vi "Untitled 1.vi"() -> ()   [LabVIEW 2015]
uses:
  <vilib>/Analysis/3filter.llb/Filter Passband Type.ctl
  <vilib>/Analysis/3filter.llb/Butterworth Filter (DBL).vi
  <vilib>/Analysis/NI_AALBase.lvlib
panel:
  in  "frequency":dbl=0.0078125 format="%0.4e"
  in  "amplitude 2":dbl=1.0 format="%0.2f"
  out "Waveform Graph":dbl[][](graph)
  out "Waveform Chart":dbl[](graph)
  in  "amplitude":dbl=1.0 format="%0.2f"
  in  "Cutoff 1":dbl=0.12500000000000006 format="%0.4f"
  in  "Cutoff 2":dbl=0.45000000000000007 format="%0.2f"
  in  "sampling freq: fs":dbl=1.0 format="%0.2f"
  in  "filter type":T1
  out "Filtered X":dbl[](array[numeric])
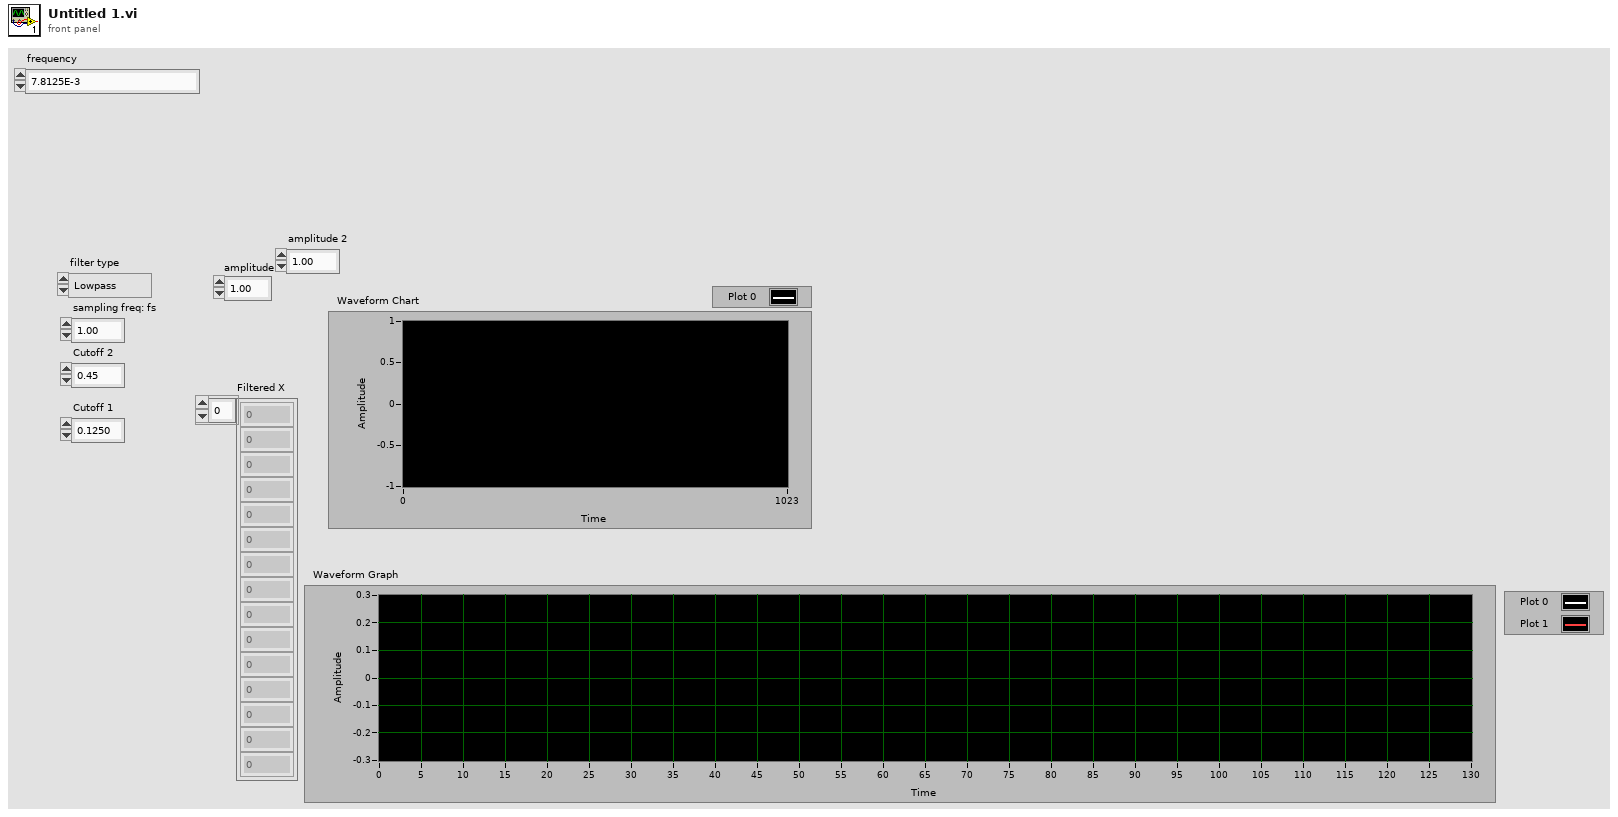
[diagram p1: front panel]
types:
  T1 = typedef "NI_AALBase.lvlib/Filter Passband Type.ctl" = enum32{"Lowpass", "Highpass", "Bandpass", "Bandstop"}
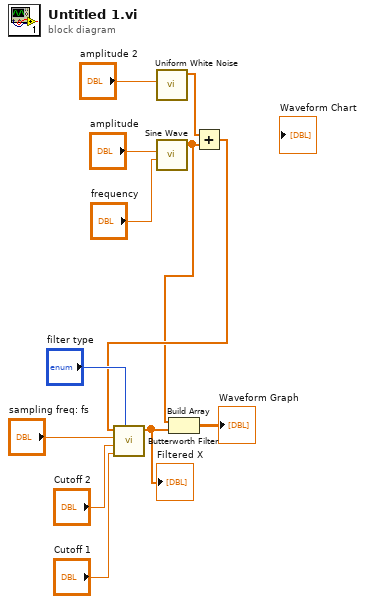
[diagram p0: block diagram]
diagram:
  n1 = call <vilib>:"Uniform White Noise.vi"("amplitude"="amplitude 2") -> ("uniform white noise"=w6:dbl[])  [unwired: 9 in, 1 out]
  n2 = call <vilib>:"Sine Wave.vi"("amplitude"="amplitude", "frequency"="frequency") -> ("sine wave"=w3:dbl[])  [unwired: 3 in, 2 out]
  n3 = Add(x=w6, y=w3) -> (x+y=w5:dbl[])
  n4 = call-poly <vilib>:"Butterworth Filter.vi"("filter type"="filter type", "low cutoff freq: fl"="Cutoff 1", "high cutoff freq: fh"="Cutoff 2", "sampling freq: fs"="sampling freq: fs", "X"=w5) -> ("Filtered X"=w8:dbl[])  [unwired: 3 in, 1 out]
  "Filtered X" <- w8
  n5 = Build Array(w3, w8) -> (→"Waveform Graph":dbl[][])
